vi "Phasor Convert (g,s) to (m, phi).vi"(2 "Phasor (g, s)":T2) -> (7 "Phasor (m, phi)":T1)   [LabVIEW 2021, in "Phasor.lvlib"]
uses:
  Phasor.lvlib
  Phasor (g, s).ctl
  Phasor (m, phi).ctl
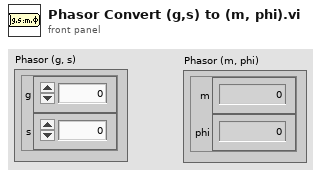
[diagram p1: front panel]
types:
  T1 = typedef "Phasor.lvlib/Phasor (m, phi).ctl" = cluster{"m":dbl, "phi":dbl}
  T2 = typedef "Phasor.lvlib/Phasor (g, s).ctl" = cluster{"g":dbl, "s":dbl}
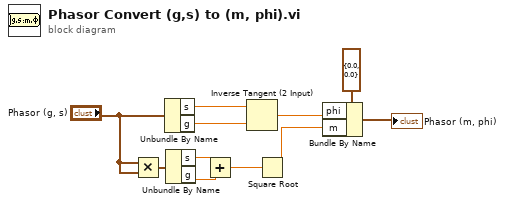
[diagram p0: block diagram]
diagram:
  n1 = Multiply(x="Phasor (g, s)", y="Phasor (g, s)") -> (x*y=w8:T2)
  n2 = Unbundle By Name("Phasor (g, s)") -> ("s"=w10:dbl, "g"=w1:dbl)
  n3 = Unbundle By Name(w8) -> ("s"=w7:dbl, "g"=w6:dbl)
  n4 = Add(x=w7, y=w6) -> (x+y=w2:dbl)
  n5 = Inverse Tangent (2 Input)(1:w1, 2:w10) -> (0:w11:dbl)
  n6 = Square Root(x=w2) -> (sqrt(x)=w5:dbl)
  n7 = Bundle By Name(cluster=T1 {"m"=0.0, "phi"=0.0} ("Phasor (m, phi)"), "phi"=w11, "m"=w5) -> (→"Phasor (m, phi)":T1)
